vi "metadata.get.vi"(8 "error in":errorcluster, 10 "Channel":refnum<class "Channel.lvclass">, 11 "Nominal Client in":refnum<class "Nominal Client.lvclass">) -> (0 "error out":errorcluster, 2 "Meta Data":T1, 3 "Nominal Client out":refnum<class "Nominal Client.lvclass">)   [LabVIEW 2020, in "Nominal Client.lvclass"]
uses:
  Nominal Client/Nominal Client.lvclass
  submodules/nominal-streaming-labview-ffi/lv_src/Channel/Channel.lvclass
  metadata.ctl
  Nominal Client/Nominal Client.lvclass/Nominal Client.ctl
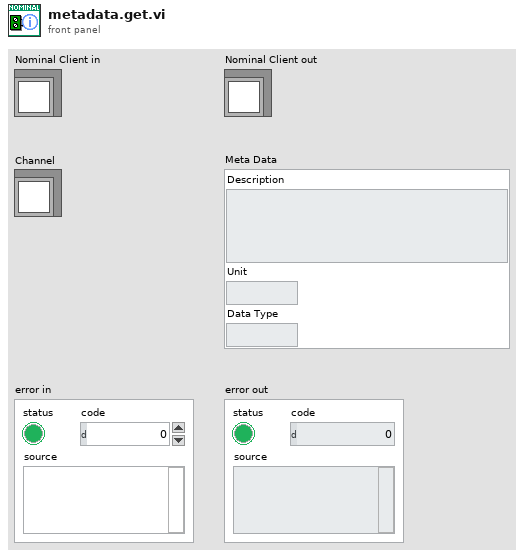
[diagram p1: front panel]
types:
  T1 = typedef "Nominal Client.lvclass/metadata.ctl" = cluster{"Description":string, "Unit":string, "Data Type":string}
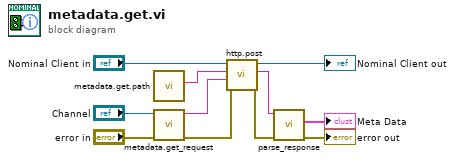
[diagram p0: block diagram]
diagram:
  n1 = call "metadata.get.path.vi"() -> ("path"=w1:string)  [unwired: 11 in]
  n2 = call "metadata.get_request.vi"("error in"="error in", "channel in"="Channel") -> ("error out"=w10:errorcluster, "JSON Payload"=w11:string)  [unwired: 8 in]
  n3 = call "http.post.vi"("error in"=w10, "Request body"=w11, "Path"=w1, "Nominal Client in"="Nominal Client in") -> ("error out"=w4:errorcluster, "Response"=w5:string, "Nominal Client out"=→"Nominal Client out":refnum<class "Nominal Client.lvclass">)  [unwired: 5 in]
  n4 = call "parse_response.vi"("error in"=w4, "Response"=w5) -> ("error out"=→"error out":errorcluster, "Meta Data"=→"Meta Data":T1)  [unwired: 8 in]
